vi "Conditional Increment - U32.vi"(2 "Condition":bool, 3 "Input":u32) -> (0 "Output":u32)   [LabVIEW 2013, in "femtoRoboLib.lvlib"]
uses:
  femtoRoboLib.lvlib
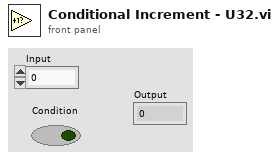
[diagram p1: front panel]
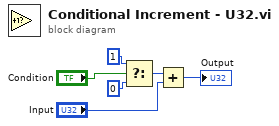
[diagram p0: block diagram]
diagram:
  n1 = Select(t=u32 1, s="Condition", f=u32 0 ("t")) -> (s? t:f=w4:u32)
  n2 = Add(x=w4, y="Input") -> (x+y=→"Output":u32)
